vi "Write Display Ref.vi"(8 "error in (no error)":errorcluster, 10 "Display Ref":refnum<vi>, 11 "Data in":refnum<class "Data.lvclass">) -> (0 "error out":errorcluster, 3 "Data out":refnum<class "Data.lvclass">)   [LabVIEW 2020, in "Data.lvclass"]
uses:
  Data.lvclass
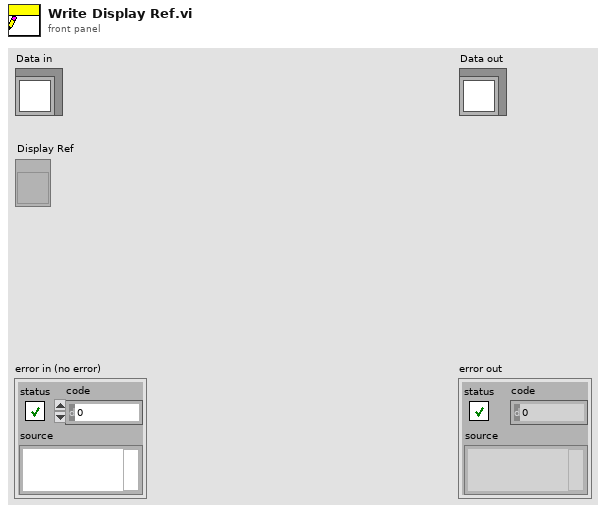
[diagram p1: front panel]
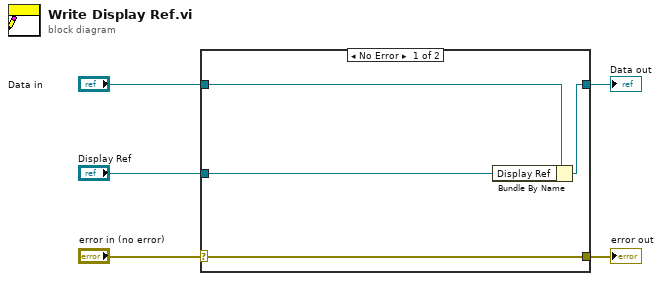
[diagram p0: block diagram]
diagram:
  n1 = case shown="No Error" "error in (no error)" {
    selector: "error in (no error)" -> [w9 w10]
    tunnel: [w9 w10] -> w4
    tunnel: [w7 w11] -> w2
    tunnel: "Data in" -> [w8 w11]
    tunnel: "Display Ref" -> [w6 _]
    frame No Error {
      n2 = Bundle By Name(cluster=w8, "Display Ref"=w6) -> (w7:refnum<class "Data.lvclass">)
    }
    frame Error {
    }
  }
  "error out" <- w4
  "Data out" <- w2
